vi "Main.vi"() -> ()   [LabVIEW 2017]
doc: "Application Simulation Interface is run to test ATM algorithms in a SW-only environment."
uses:
  View Model/Controls/Interface.ctl
panel:
  out "error out":errorcluster
  in  "error in (no error)":errorcluster
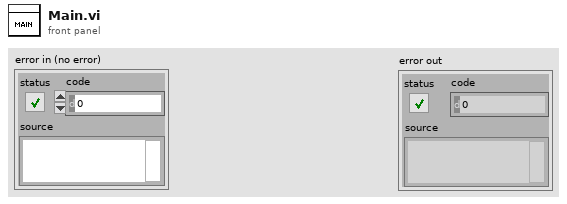
[diagram p1: front panel]
types:
  T1 = typedef "View Model.ctl" = cluster{"Error Model":T2, "Shared Model":T3, "Config Model":T4, "Controller Model":T5}
  T2 = typedef "Error Model.ctl" = cluster{"Error Event":refnum<user-event>}
  T3 = typedef "Shared Model.ctl" = cluster{"Stop Event":refnum<user-event>, "Stop DVR":refnum<data-value>}
  T4 = typedef "Config Model.ctl" = cluster{"Config CMD":refnum<user-event>, "Config Data DVR":refnum<data-value>}
  T5 = typedef "Controller Model.ctl" = cluster{"Controller Overhead DVR":refnum<data-value>, "Deposit Received Change":refnum<user-event>, "Fund Transaction Change":refnum<user-event>, "Card Read Change":refnum<user-event>, "Controller CMD Change":refnum<user-event>, "Transaction Change":refnum<user-event>, "Keypad Change":refnum<user-event>, "Message Change":refnum<user-event>}
  T6 = typedef "Interface.ctl" = enum16{"Simulated", "Physical"}
  T7 = enum32{"invalid app kind", "Development System", "Run Time System", "Student Edition", "Embedded LabVIEW", "Evaluation", "Custom"}
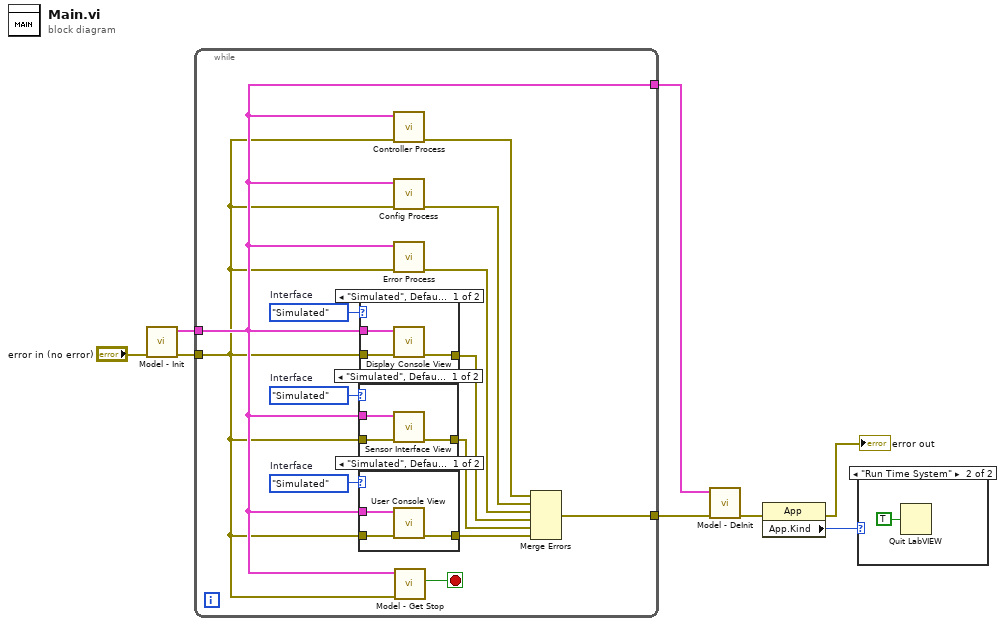
[diagram p0: block diagram]
diagram:
  n1 = call "Model - Init.vi"("error in (no error)"="error in (no error)") -> ("error out"=w7:errorcluster, "View Model"=w6:T1)  [unwired: 9 in]
  n2 = while {
    tunnel: w7 -> [w10]
    tunnel: w6 -> [w11]
    tunnel: [w12] -> w5
    tunnel: [w11] -> w4
    stop <- w9 stop-if-true
    w19 = Interface."Simulated"  # Interface
    w20 = Interface."Simulated"  # Interface
    w21 = Interface."Simulated"  # Interface
    n3 = case shown="\"Simulated\", Default" w20 {
      tunnel: w11 -> [w28 _]
      tunnel: w10 -> [w27 w29]
      tunnel: [w26 w29] -> w17
      frame "Simulated", Default {
        n4 = call "Sensor Interface View.vi"("error in (no error)"=w27, "View Model"=w28) -> ("error out"=w26:errorcluster)  [unwired: 9 in]
      }
      frame "Physical" {
      }
    }
    n5 = case shown="\"Simulated\", Default" w19 {
      tunnel: w11 -> [w24 _]
      tunnel: w10 -> [w23 w25]
      tunnel: [w22 w25] -> w18
      frame "Simulated", Default {
        n6 = call "User Console View.vi"("error in (no error)"=w23, "View Model"=w24) -> ("error out"=w22:errorcluster)  [unwired: 9 in]
      }
      frame "Physical" {
      }
    }
    n7 = case shown="\"Simulated\", Default" w21 {
      tunnel: w10 -> [w32 w33]
      tunnel: w11 -> [w31 _]
      tunnel: [w30 w33] -> w16
      frame "Simulated", Default {
        n8 = call "Display Console View.vi"("error in (no error)"=w32, "View Model"=w31) -> ("error out"=w30:errorcluster)  [unwired: 9 in]
      }
      frame "Physical" {
      }
    }
    n9 = call "Controller Process.vi"("error in (no error)"=w10, "View Model"=w11) -> ("error out"=w13:errorcluster)  [unwired: 9 in]
    n10 = call "Config Process.vi"("error in (no error)"=w10, "View Model"=w11) -> ("error out"=w14:errorcluster)  [unwired: 8 in, 1 out]
    n11 = call "Error Process.vi"("error in (no error)"=w10, "View Model"=w11) -> ("error out"=w15:errorcluster)  [unwired: 8 in, 1 out]
    n12 = call "Model - Get Stop.vi"("error in (no error)"=w10, "View Model"=w11) -> ("Stop"=w9:bool)  [unwired: 7 in, 2 out]
    n13 = Merge Errors(w13, w14, w15, w16, w17, w18) -> (w12:errorcluster)
  }
  n14 = call "Model - DeInit.vi"("error in (no error)"=w5, "View Model"=w4) -> ("error out"=w3:errorcluster)  [unwired: 9 in]
  n15 = property class="App"(error in=w3) -> (error out=→"error out":errorcluster, "App.Kind"=w2:T7)  [unwired: 1 in, 1 out]
  n16 = case shown="\"Run Time System\"" w2 {
    frame "Development System", Default {
    }
    frame "Run Time System" {
      n17 = Quit LabVIEW(quit? (T)=TRUE) -> ()
    }
  }
